vi "PulseWidth.vi"(0 "Column Definitions 2":T1(array[cluster]) {"Offset" format="%.2f"; "Resolution" format="%.2f"}, 1 "error in":errorcluster) -> (2 "Pulse Width Cluster":cluster{dbl, dbl}, 4 "error out":errorcluster)   [LabVIEW 2009]
uses:
  Acquisition Settings.vi
panel:
  out "element 2":dbl
  out "element":dbl
  out "x*y":dbl
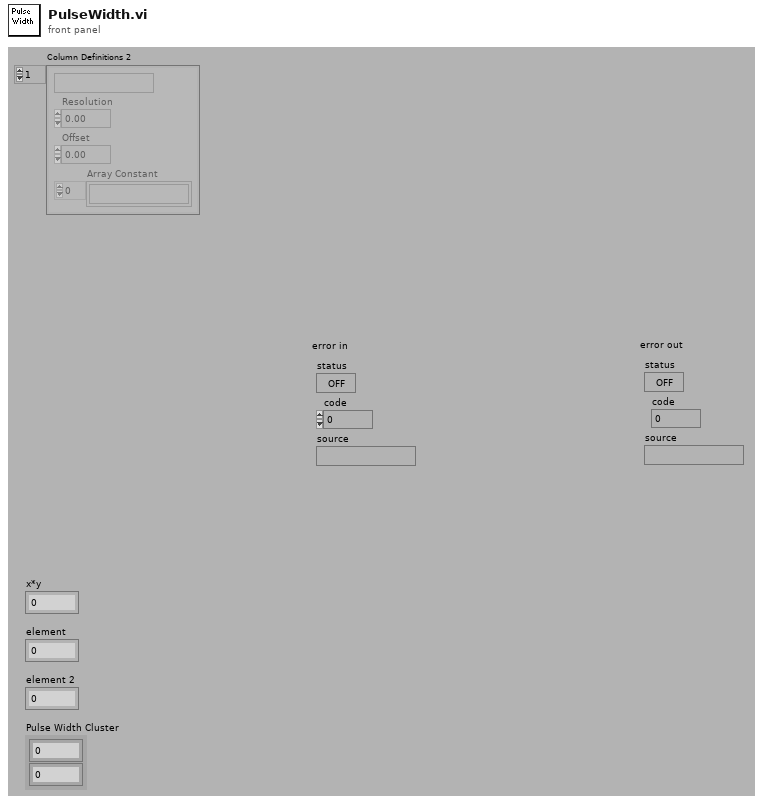
[diagram p1: front panel]
types:
  T1 = cluster{string, "Resolution":dbl, "Offset":dbl, "Array Constant":string[]}[]
  T2 = cluster{"Name":string, "Device Number":i16, "Counter Number":i16, "Pulse Spec 1 (Clocks)":u32, "Pulse Spec 2 (Clocks)":u32, "Signal Routing Configuration":i16, "Inverted":bool}[]
  T3 = cluster{string, "Resolution":dbl, "Offset":dbl, "Array Constant":string[]}
  T4 = cluster{"Name":string, "Device Number":i16, "Counter Number":i16, "Pulse Spec 1 (Clocks)":u32, "Pulse Spec 2 (Clocks)":u32, "Signal Routing Configuration":i16, "Inverted":bool}
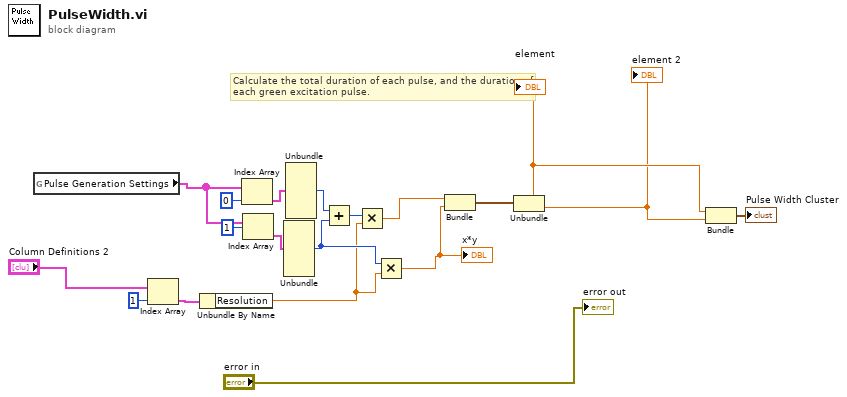
[diagram p0: block diagram]
diagram:
  # "Calculate the total duration of each pulse, and the duration of \neach green excitation pulse."
  n1 = global read "Acquisition Settings.vi" "Pulse Generation Settings"() -> (w16:T2)
  n2 = Index Array(array="Column Definitions 2", index=1 ("Index")) -> (element=w11:T3)
  n3 = Unbundle By Name(w11) -> ("Resolution"=w9:dbl)
  n4 = Index Array(array=w16, index=0) -> (element=w18:T4)
  n5 = Index Array(array=w16, index=1) -> (element=w15:T4)
  n6 = Unbundle(w15) -> ("Pulse Spec 1 (Clocks)"=w10:u32)  [unwired: 6 out]
  n7 = Unbundle(w18) -> ("Pulse Spec 1 (Clocks)"=w14:u32)  [unwired: 6 out]
  n8 = Add(x=w14, y=w10) -> (x+y=w13:u32)
  n9 = Multiply(x=w13, y=w9) -> (x*y=w5:dbl)
  n10 = Multiply(x=w10, y=w9) -> (x*y=w6:dbl)
  "x*y" <- w6
  n11 = Bundle(w5, w6) -> (w4:cluster{dbl, dbl})  [unwired: 1 in]
  n12 = Unbundle(w4) -> (w3:dbl, w2:dbl)
  "element" <- w3
  "element 2" <- w2
  n13 = Bundle(w3, w2) -> (→"Pulse Width Cluster":cluster{dbl, dbl})  [unwired: 1 in]
  "error out" <- "error in"
